vi "Check Double Click Top level.vi"(8 "error in (no error)":errorcluster, 11 "path":path) -> (0 "error out":errorcluster, 2 "Number of Peaks":i32, 3 "Peak Indexes":i32[](array[numeric]), 4 "Y":dbl[](graph), 6 "Waveform Graph":waveform(dbl)(graph))   [LabVIEW 2019]
uses:
  <vilib>/measure/maresamp.llb/Resample Waveform (single shot).vi
  <vilib>/measure/NI_MAPro.lvlib
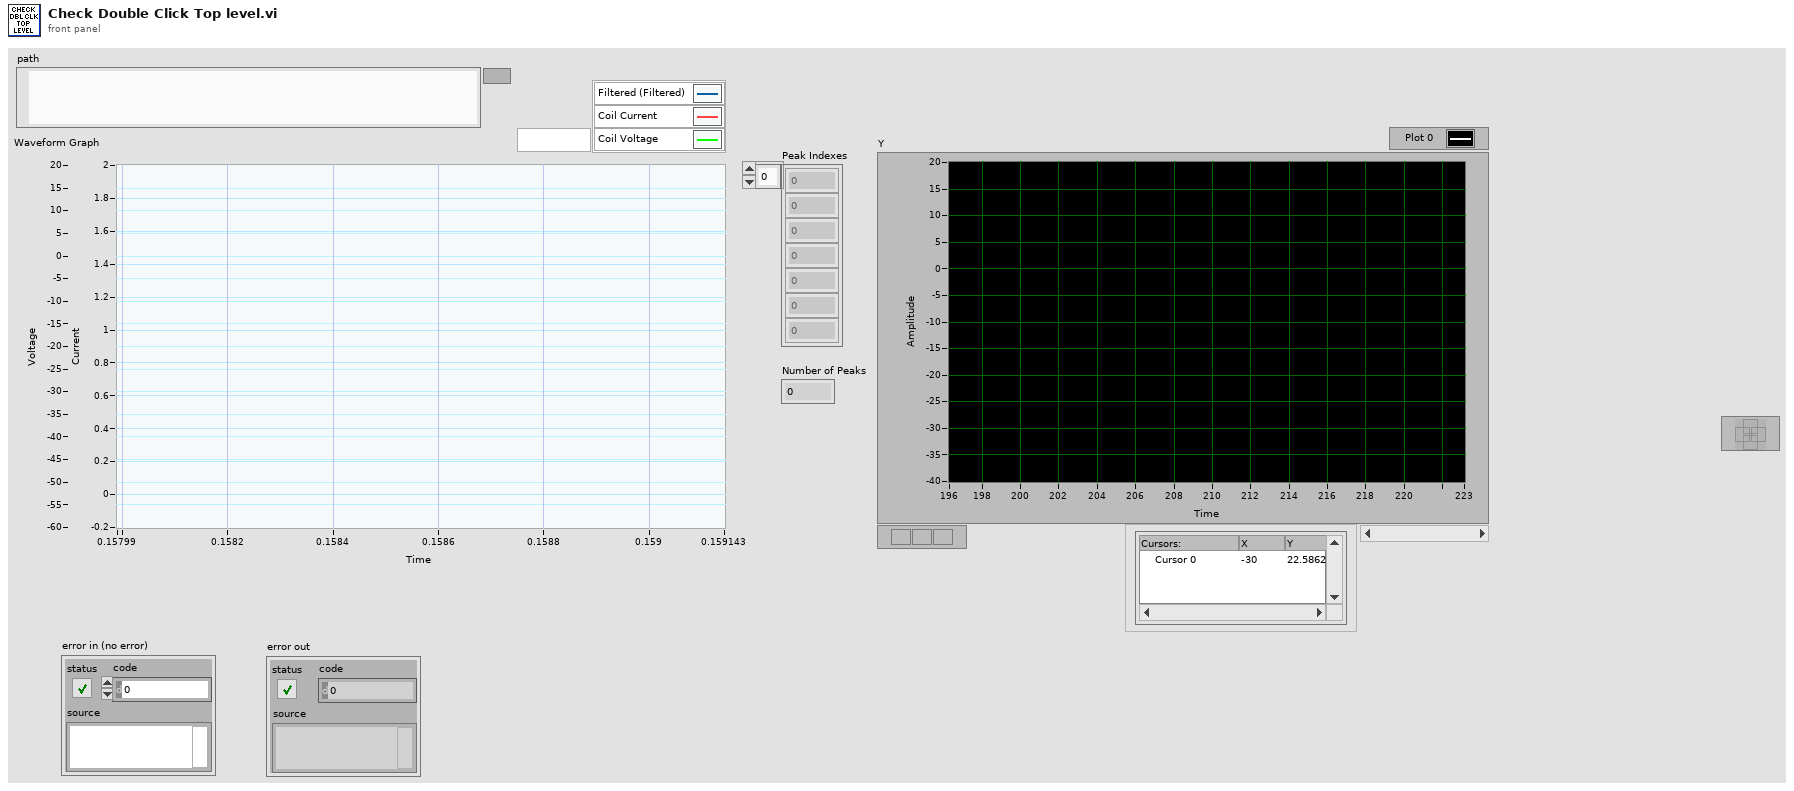
[diagram p1: front panel]
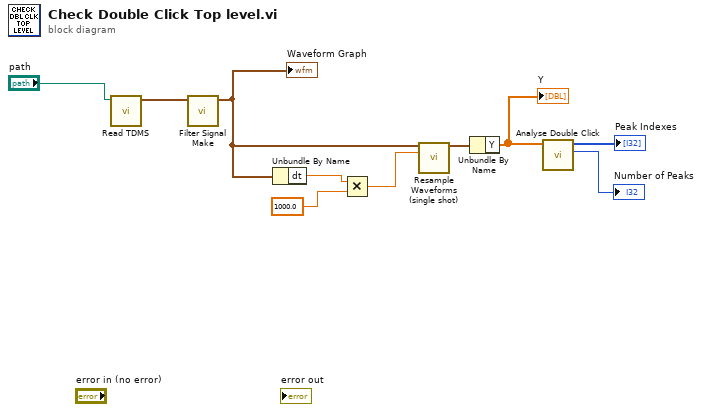
[diagram p0: block diagram]
diagram:
  n1 = call "Read TDMS.vi"("file path"="path") -> ("Waveform Graph"=w1:waveform(dbl)[])  [unwired: 9 in, 1 out]
  n2 = call "Filter Signal Make.vi"("PASS DC 12V"=w1) -> ("Filter + Smooth"=w3:waveform(dbl))  [unwired: 8 in, 2 out]
  "Waveform Graph" <- w3
  n3 = Unbundle By Name(w3) -> ("dt"=w4:dbl)
  n4 = Multiply(x=w4, y=1000.0) -> (x*y=w6:dbl)
  n5 = call-poly <vilib>:"Resample Waveforms (single shot).vi"("waveform in"=w3, "dt"=w6) -> ("resampled waveform out"=w8:waveform(dbl))  [unwired: 10 in, 3 out]
  n6 = Unbundle By Name(w8) -> ("Y"=w9:dbl[])
  "Y" <- w9
  n7 = call "Analyse Double Click.vi"("Waveform in"=w9) -> ("Number of Valleys"=→"Number of Peaks":i32, "Valley Indexes"=→"Peak Indexes":i32[])  [unwired: 8 in, 1 out]
